vi "Increment.vi"(8 "error in (no error)":errorcluster, 10 "Amount":i32, 11 "FirstAF in":refnum<class "FirstAF.lvclass">) -> (0 "error out":errorcluster, 3 "FirstAF out":refnum<class "FirstAF.lvclass">)   [LabVIEW 2019, in "FirstAF.lvlib" / "FirstAF.lvclass"]
uses:
  FirstAF.lvclass
  FirstAF.lvclass/FirstAF.ctl
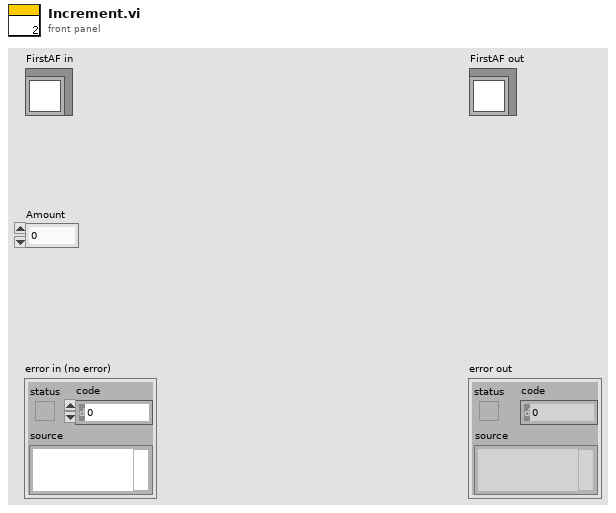
[diagram p1: front panel]
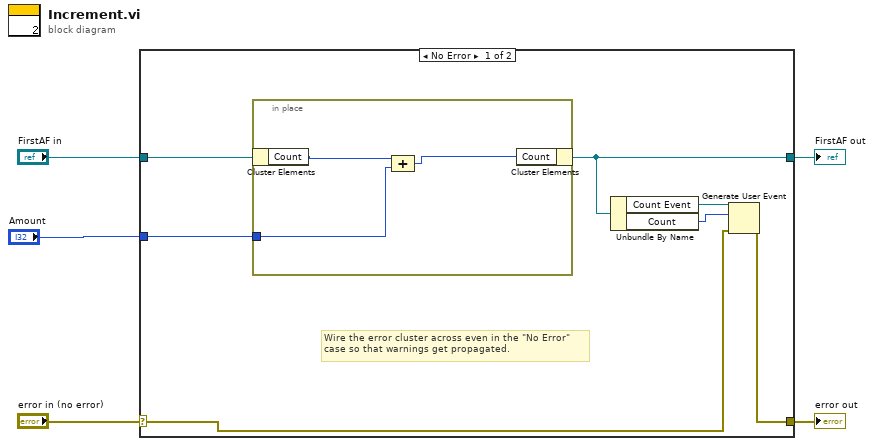
[diagram p0: block diagram]
diagram:
  n1 = case shown="No Error" "error in (no error)" {
    selector: "error in (no error)" -> [w7 w17]
    tunnel: [w6 w17] -> w4
    tunnel: [w10 w16] -> w2
    tunnel: "FirstAF in" -> [w12 w16]
    tunnel: "Amount" -> [w11 _]
    frame No Error {
      # "Wire the error cluster across even in the \"No Error\"\ncase so that warnings get propagated."
      n2 = in-place {
        in-place-border: w11 -> [w13]
        n3 = in-place-cluster #1(w12) -> ("Count"=w15:i32)
        n4 = Compound Arithmetic op=ADD(w15, w13) -> (w14:i32)
        n5 = in-place-cluster #1("Count"=w14) -> (w10:refnum<class "FirstAF.lvclass">)
      }
      n6 = Unbundle By Name(w10) -> ("Count Event"=w9:refnum<user-event>, "Count"=w8:i32)
      n7 = Generate User Event(user event=w9, event data cluster=w8, error in=w7) -> (error out=w6:errorcluster)  [unwired: 1 in, 1 out]
    }
    frame Error {
    }
  }
  "error out" <- w4
  "FirstAF out" <- w2
